vi "Main VI.vi"(11 "Error In":errorcluster) -> (15 "Error Out":errorcluster)   [LabVIEW 2020, in "DNL INL Test.lvlib"]
uses:
  DNL INL Test.lvlib
  Typedef/Queue Operation.ctl
  Typedef/Data Line.ctl
  Class/INL DNL Test/Test/Parent/Test.lvclass
  Typedef/User event controls.ctl
  Class/INL DNL Test/Test/Children/INL DNL Test/INL DNL Test.lvclass
  D:/SDLC/Class/INL DNL Test/Test/Parent/Test.lvclass
  Class/INL DNL Test/Device/Parent/Device.lvclass
panel:
  in  "Calculate":bool
  in  "Available Test":string(tree)
  out "Graph Pic":picture
  out "Config Pic":picture
  out "Mode Pic":picture
  out "Home Pic":picture
  in  "Status and graph":bool
  in  "Configuration":bool
  in  "Mode selection":bool
  in  "Home":bool
  out "Status":string
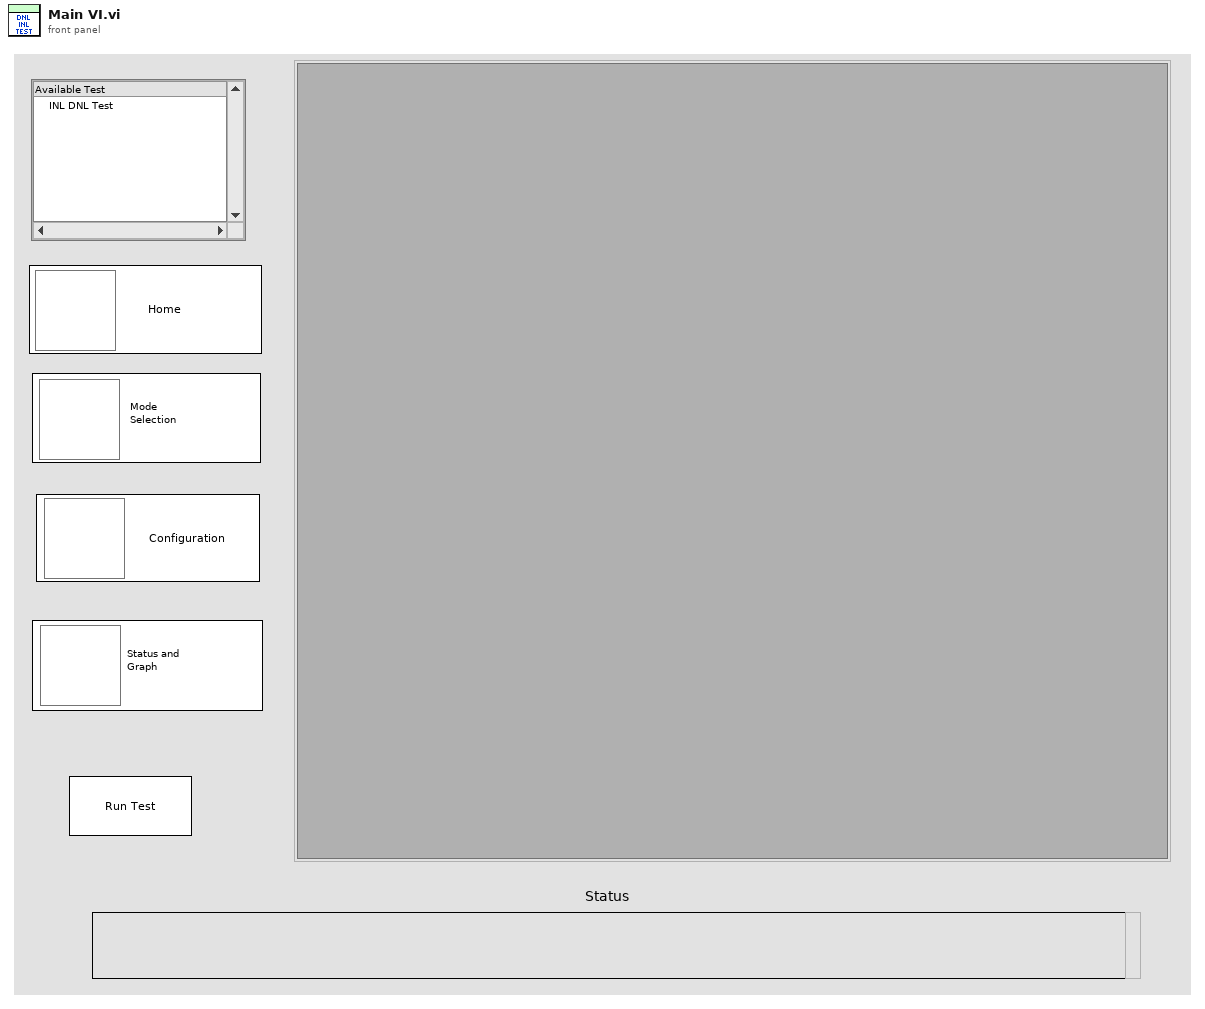
[diagram p1: front panel]
types:
  T1 = typedef "DNL INL Test.lvlib/Data Line.ctl" = cluster{"DVR":refnum<data-value>, "Subpanel Ref":refnum<vi>, "Class Selected?":bool, "Status Msg":string, "Test Name":string, "Status":string, "Mode Ref":refnum<vi>, "Config Ref":refnum<vi>}
  T2 = typedef "DNL INL Test.lvlib/Queue Operation.ctl" = enum16{"Create Queue", "Enqueue", "Dequeue", "Enstack", "Flush Queue", "Release Queue"}
  T3 = typedef "DNL INL Test.lvlib/User event controls.ctl" = enum16{"Create", "Generate", "Get Ref", "Destroy"}
  T4 = typedef "imagedata.ctl" = cluster{"image type":i32, "image depth":i32, "image":u8[], "mask":u8[], "colors":u32[], "Rectangle":cluster{"left":i16, "top":i16, "right":i16, "bottom":i16}}
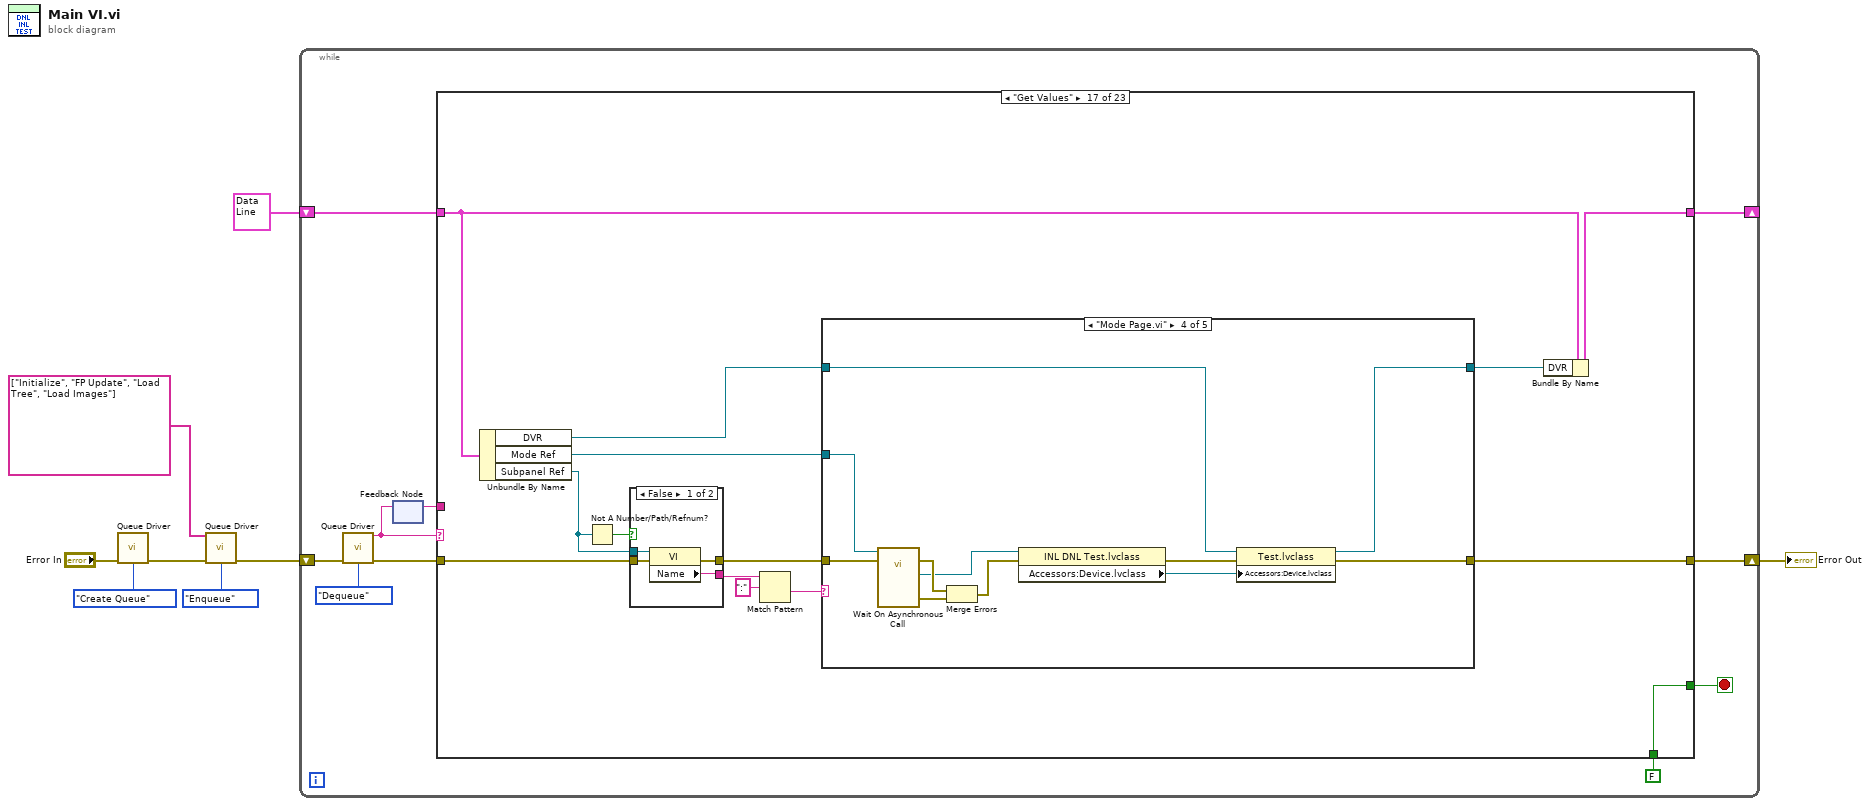
[diagram p0: block diagram]
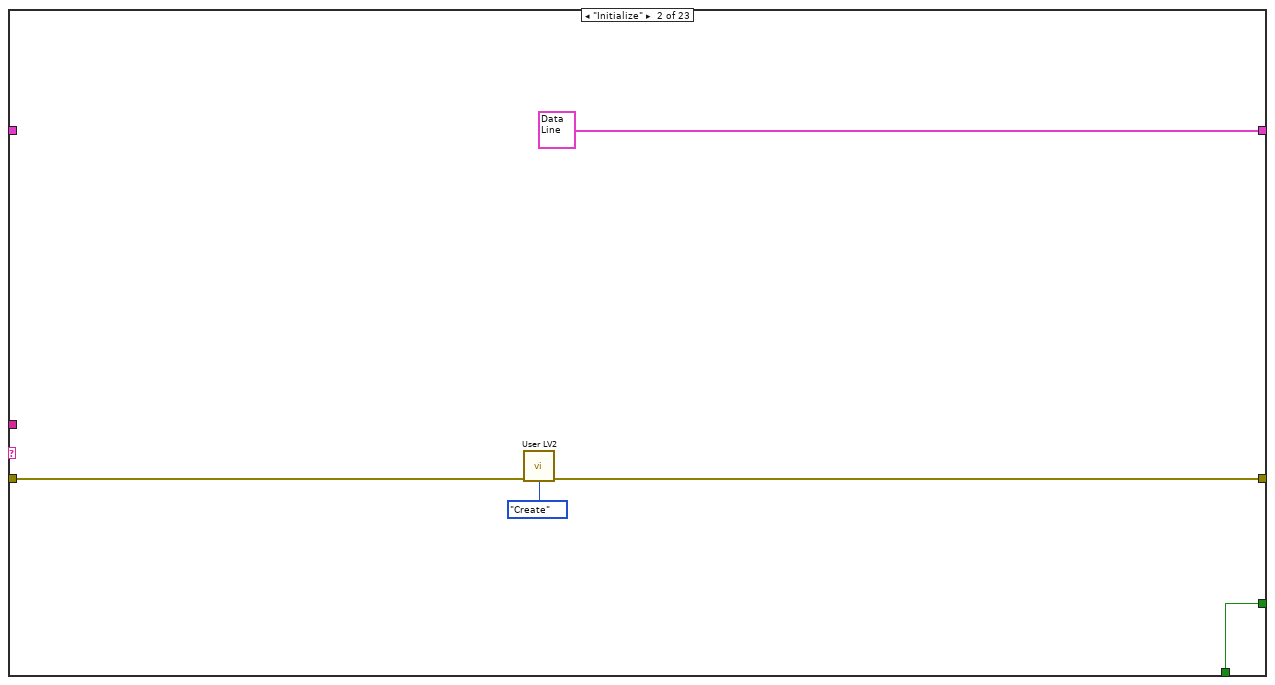
[diagram p3: hidden frame]
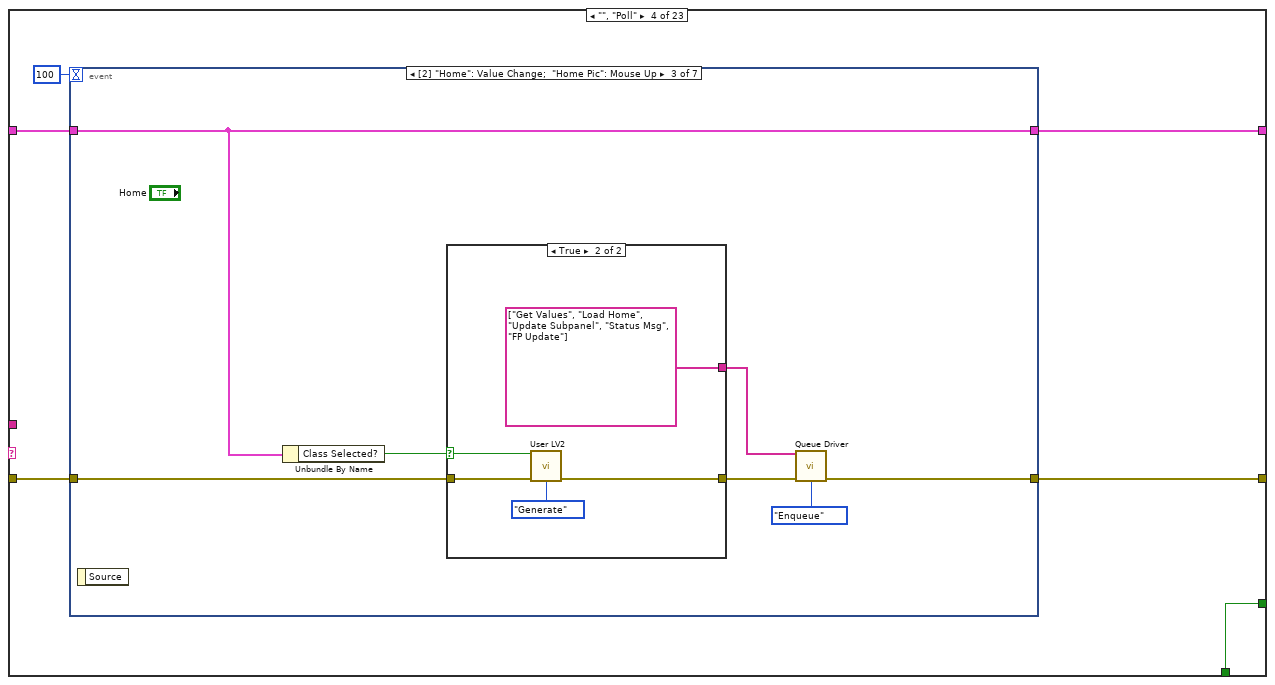
[diagram p5: hidden frame]
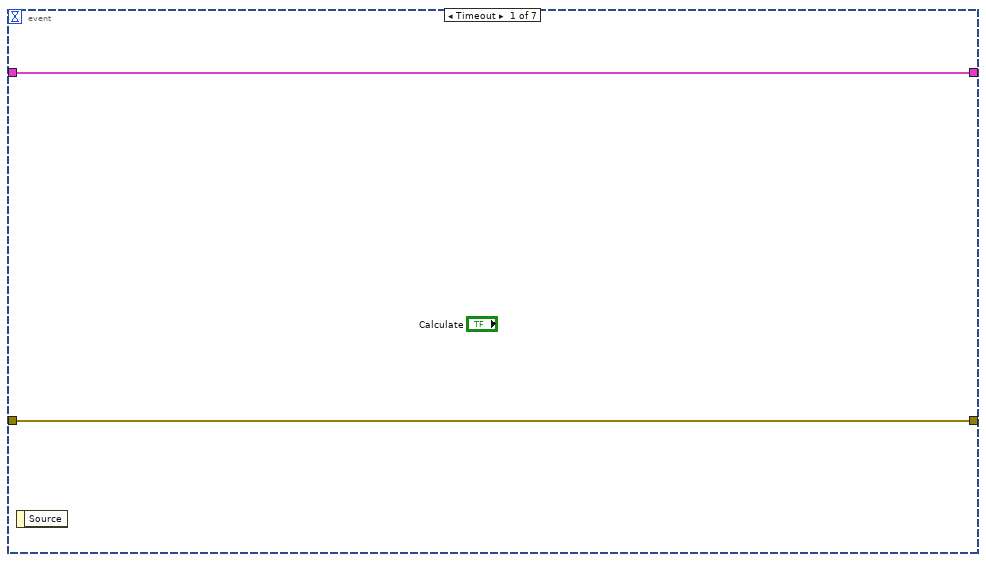
[diagram p6: hidden frame]
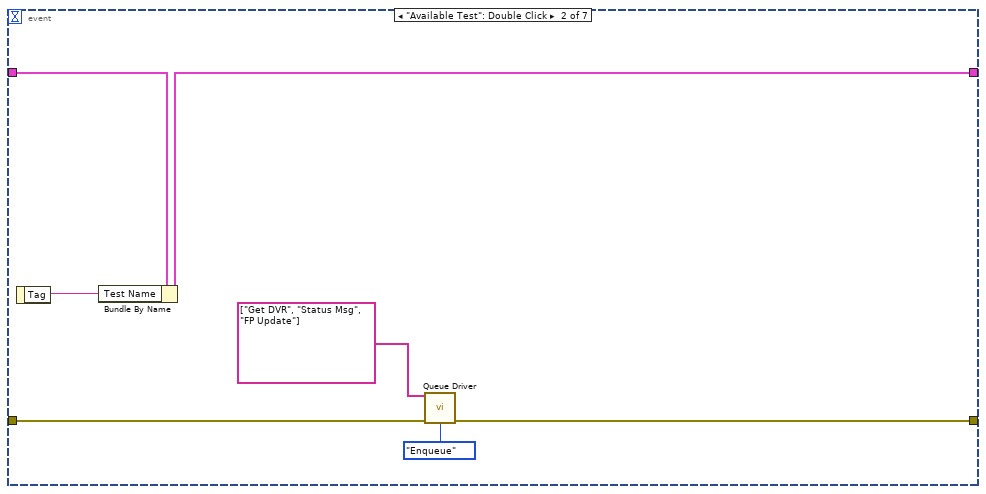
[diagram p7: hidden frame]
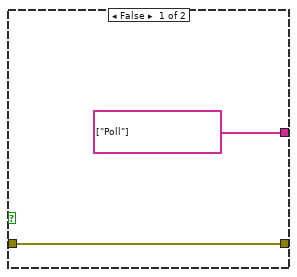
[diagram p8: hidden frame]
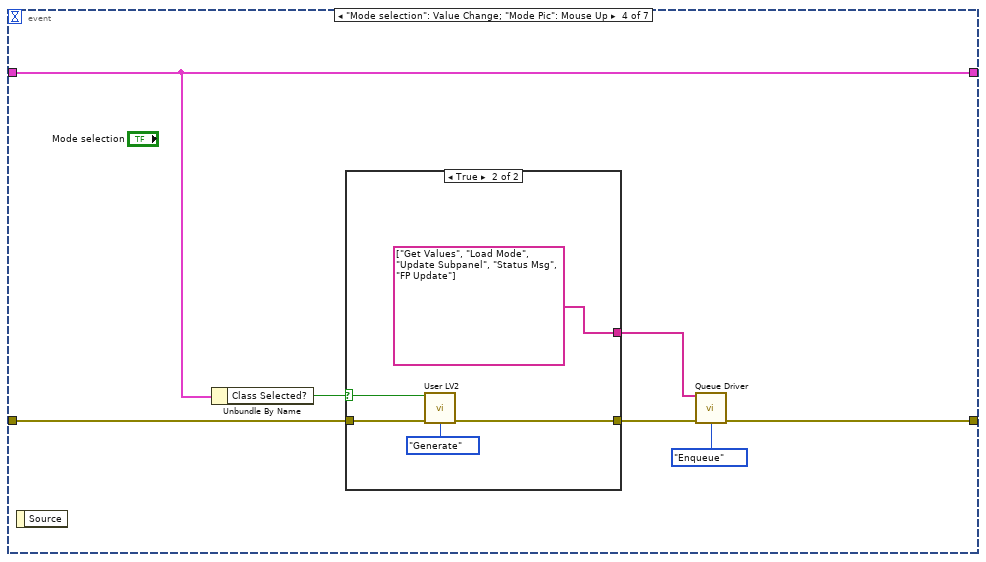
[diagram p9: hidden frame]
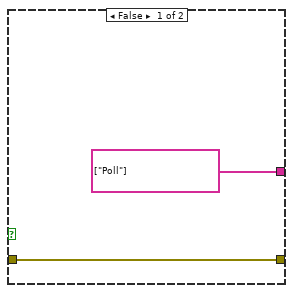
[diagram p10: hidden frame]
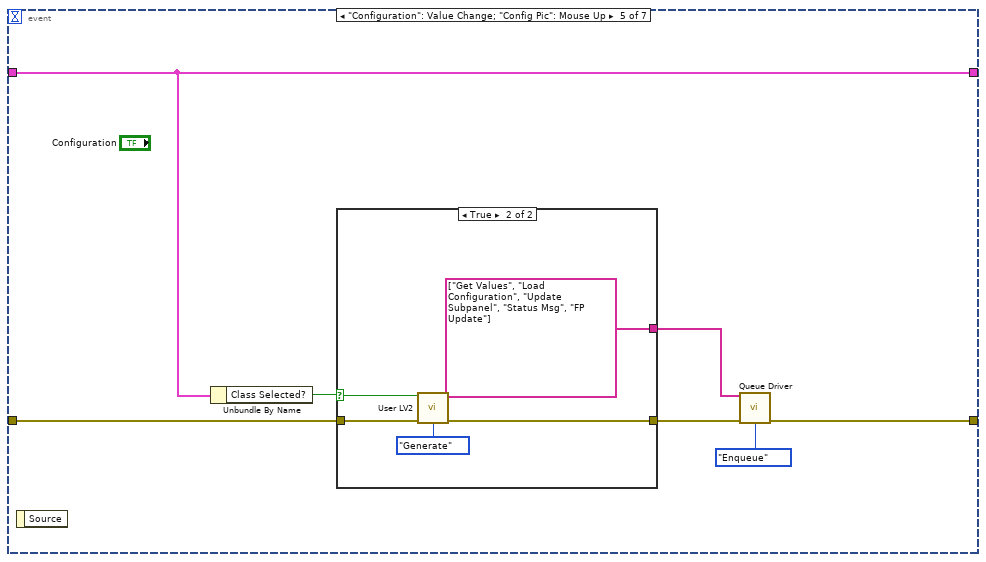
[diagram p11: hidden frame]
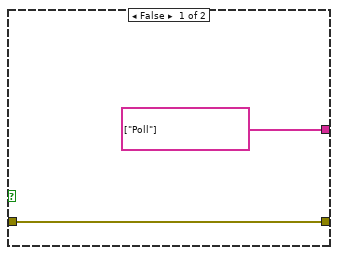
[diagram p12: hidden frame]
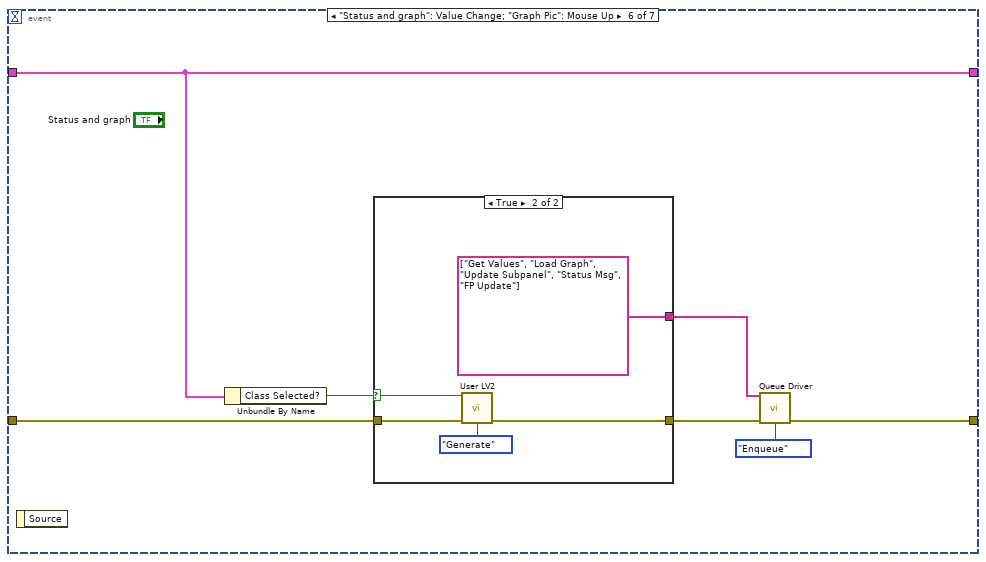
[diagram p13: hidden frame]
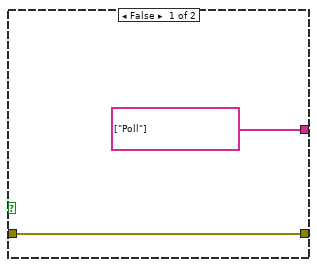
[diagram p14: hidden frame]
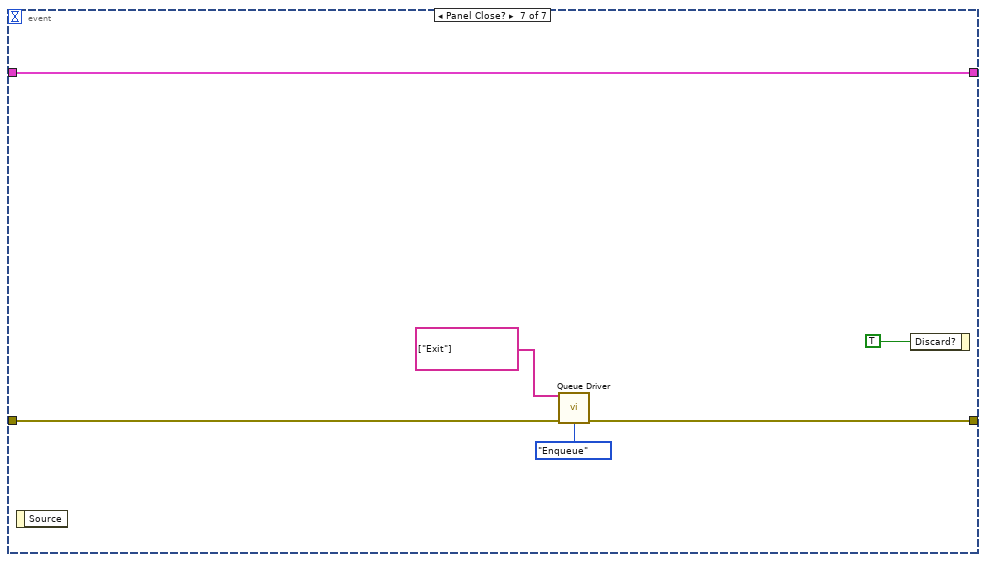
[diagram p15: hidden frame]
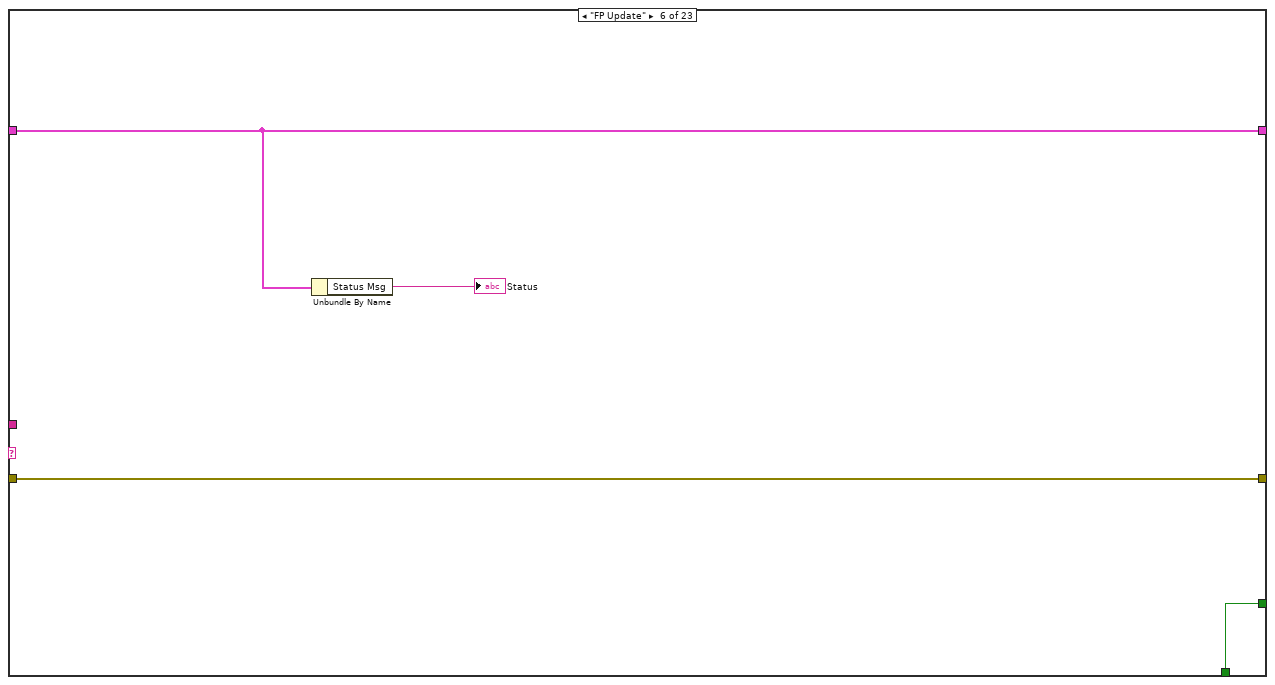
[diagram p17: hidden frame]
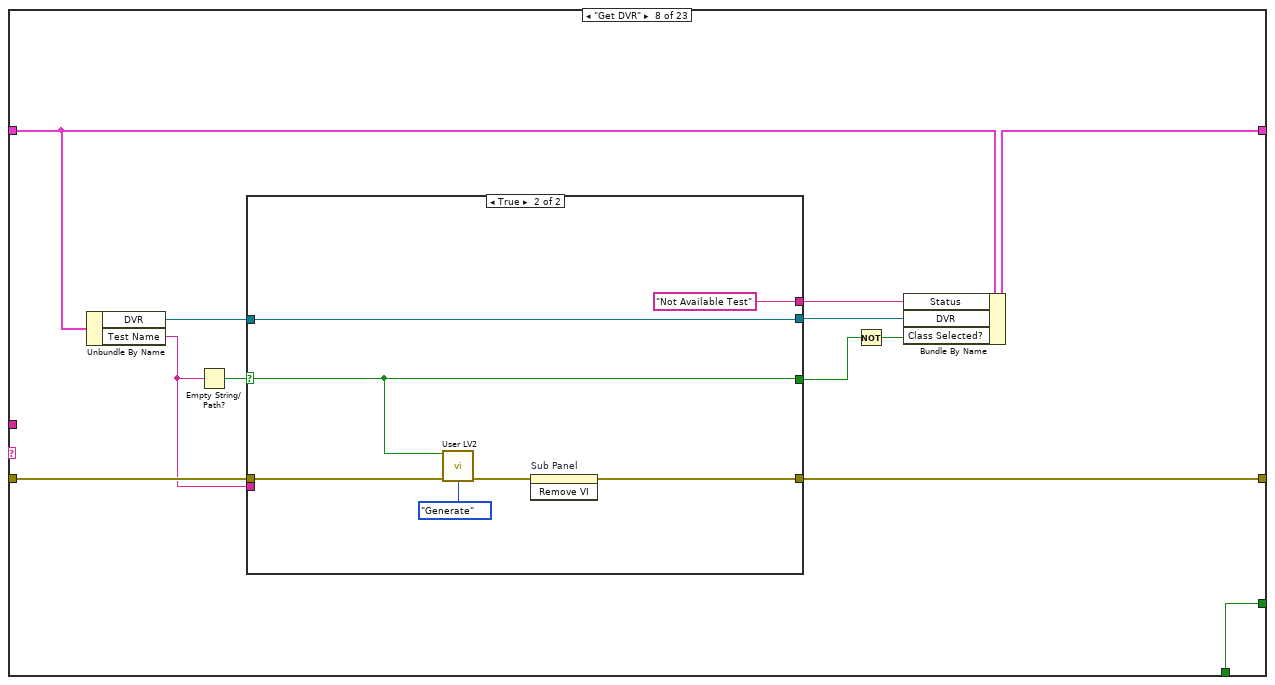
[diagram p19: hidden frame]
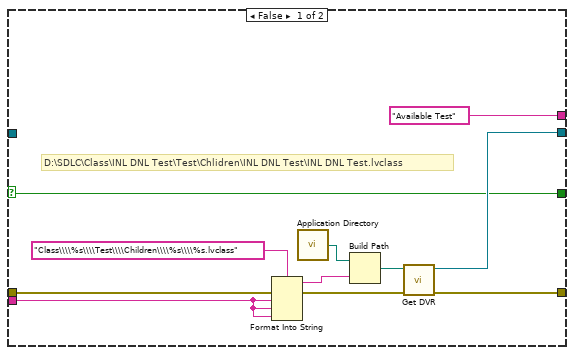
[diagram p20: hidden frame]
diagram:
  n1 = call "Queue Driver.vi"("Error In"="Error In", "Queue Operation"=Queue_Operation."Create Queue") -> ("Error Out"=w6:errorcluster)  [unwired: 12 in, 1 out]
  n2 = call "Queue Driver.vi"("States"=string[] ["Initialize", "FP Update", "Load Tree", "Load Images"], "Error In"=w6, "Queue Operation"=Queue_Operation."Enqueue") -> ("Error Out"=w3:errorcluster)  [unwired: 11 in, 1 out]
  n3 = while {
    shift-right: [w13] -> w2
    shift-left: w3 -> [w18]
    shift-right: [w9] -> _
    shift-left: T1 {"DVR"=refnum, "Subpanel Ref"=refnum, "Class Selected?"=FALSE, "Status Msg"="", "Test Name"="", "Status"="", "Mode Ref"=refnum, "Config Ref"=refnum} ("Data Line") -> [w10]
    stop <- w11 stop-if-true
    n4 = call "Queue Driver.vi"("Error In"=w18, "Queue Operation"=Queue_Operation."Dequeue") -> ("Dequeue Element"=w16:string, "Error Out"=w14:errorcluster)  [unwired: 12 in]
    n5 = feedback-in #1(w16) -> ()
    n6 = feedback #1() -> (w15:string)  [unwired: 1 in]
    n7 = case shown="\"Get Values\"" w16 {
      selector: w16 -> [_ _ _ _ _ _ _ _ _ _ _ _ _ _ _ _ _ _ _ _ _ _ w378]
      tunnel: w15 -> [_ _ _ _ _ _ _ _ _ _ _ _ _ _ _ _ _ _ w342 _ _ _ _]
      tunnel: w14 -> [w21 w26 w29 w35 w109 w113 w116 w127 w153 w182 w184 w200 w209 w219 w224 w233 w296 w325 w345 w348 w364 w367 w381]
      tunnel: [w21 w24 w29 w34 w109 w113 w116 w126 w151 w182 w190 w193 w208 w214 w221 w232 w295 w325 w332 w348 w360 w367 w369] -> w13
      tunnel: FALSE -> [w20 w25 w28 w32 w108 w112 w115 w128 w158 w181 w191 w201 w211 w220 w225 w234 w297 w324 w326 w347 _ w366 w382]
      tunnel: [w20 w25 w28 w32 w108 w112 w115 w128 w158 w181 w191 w201 w211 w220 w225 w234 w297 w324 w326 w347 TRUE ("T button?") w366 w382] -> w11
      tunnel: w10 -> [w19 _ w27 w31 w107 w111 w114 w121 w157 w180 w188 w198 w207 w217 w223 w228 w286 w323 w329 w346 w353 w365 w368]
      tunnel: [w19 T1 {"DVR"=refnum, "Subpanel Ref"=refnum, "Class Selected?"=FALSE, "Status Msg"="", "Test Name"="", "Status"="", "Mode Ref"=refnum, "Config Ref"=refnum} ("Data Line") w27 w30 w107 w111 w114 w120 w157 w180 w185 w196 w204 w213 w223 w226 w284 w323 w327 w346 w353 w365 w368] -> w9
      frame "/****Initialize****/" {
      }
      frame "Initialize" {
        n8 = call "User LV2.vi"("Error In"=w26, "User event controls"=User_event_controls."Create") -> ("Error Out"=w24:errorcluster)  [unwired: 12 in, 1 out]
      }
      frame "/****User inputs****/" {
      }
      frame "", "Poll" {
        n9 = event shown="[2] \"Home\": Value Change;  \"Home Pic\": Mouse Up" {
          selector: _ -> [_ _ _ _ _ _ _]
          dyn-events: _ -> [_ _ _ _ _ _ _]
          timeout: 100 -> [_ _ _ _ _ _ _]
          tunnel: w35 -> [w37 w41 w48 w62 w76 w90 w104]
          tunnel: [w37 w40 w51 w63 w77 w91 w103] -> w34
          tunnel: w31 -> [w36 w44 w46 w60 w74 w88 w106]
          tunnel: [w36 w43 w46 w60 w74 w88 w106] -> w30
          event Timeout {
            n10 = event-data() -> ()  [unwired: 1 in, 1 out]
          }
          event "Available Test": Double Click {
            n11 = event-data() -> ("Tag"=w42:string)  [unwired: 1 in]
            n12 = Bundle By Name(cluster=w44, "Test Name"=w42) -> (w43:T1)
            n13 = call "Queue Driver.vi"("States"=string[] ["Get DVR", "Status Msg", "FP Update"], "Error In"=w41, "Queue Operation"=Queue_Operation."Enqueue") -> ("Error Out"=w40:errorcluster)  [unwired: 11 in, 1 out]
          }
          event "Home": Value Change; "Home Pic": Mouse Up {
            n14 = event-data() -> ()  [unwired: 1 in, 1 out]
            n15 = Unbundle By Name(w46) -> ("Class Selected?"=w45:bool)
            n16 = case shown="True" w45 {
              selector: w45 -> [_ w54]
              tunnel: [string[] ["Poll"] ("States") string[] ["Get Values", "Load Home", "Update Subpanel", "Status Msg", "FP Update"] ("States")] -> w49
              tunnel: w48 -> [w52 w57]
              tunnel: [w52 w56] -> w47
              frame False {
              }
              frame True {
                n17 = call "User LV2.vi"("Stop"=w54, "Error In"=w57, "User event controls"=User_event_controls."Generate") -> ("Error Out"=w56:errorcluster)  [unwired: 11 in, 1 out]
              }
            }
            n18 = call "Queue Driver.vi"("States"=w49, "Error In"=w47, "Queue Operation"=Queue_Operation."Enqueue") -> ("Error Out"=w51:errorcluster)  [unwired: 11 in, 1 out]
          }
          event "Mode selection": Value Change; "Mode Pic": Mouse Up {
            n19 = event-data() -> ()  [unwired: 1 in, 1 out]
            n20 = Unbundle By Name(w60) -> ("Class Selected?"=w59:bool)
            n21 = case shown="True" w59 {
              selector: w59 -> [_ w68]
              tunnel: [string[] ["Poll"] ("States") string[] ["Get Values", "Load Mode", "Update Subpanel", "Status Msg", "FP Update"] ("States")] -> w64
              tunnel: [w66 w70] -> w61
              tunnel: w62 -> [w66 w72]
              frame False {
              }
              frame True {
                n22 = call "User LV2.vi"("Stop"=w68, "Error In"=w72, "User event controls"=User_event_controls."Generate") -> ("Error Out"=w70:errorcluster)  [unwired: 11 in, 1 out]
              }
            }
            n23 = call "Queue Driver.vi"("States"=w64, "Error In"=w61, "Queue Operation"=Queue_Operation."Enqueue") -> ("Error Out"=w63:errorcluster)  [unwired: 11 in, 1 out]
          }
          event "Configuration": Value Change; "Config Pic": Mouse Up {
            n24 = event-data() -> ()  [unwired: 1 in, 1 out]
            n25 = Unbundle By Name(w74) -> ("Class Selected?"=w73:bool)
            n26 = case shown="True" w73 {
              selector: w73 -> [_ w82]
              tunnel: [string[] ["Poll"] ("States") string[] ["Get Values", "Load Configuration", "Update Subpanel", "Status Msg", "FP Update"] ("States")] -> w78
              tunnel: w76 -> [w80 w86]
              tunnel: [w80 w84] -> w75
              frame False {
              }
              frame True {
                n27 = call "User LV2.vi"("Stop"=w82, "Error In"=w86, "User event controls"=User_event_controls."Generate") -> ("Error Out"=w84:errorcluster)  [unwired: 11 in, 1 out]
              }
            }
            n28 = call "Queue Driver.vi"("States"=w78, "Error In"=w75, "Queue Operation"=Queue_Operation."Enqueue") -> ("Error Out"=w77:errorcluster)  [unwired: 11 in, 1 out]
          }
          event "Status and graph": Value Change; "Graph Pic": Mouse Up {
            n29 = event-data() -> ()  [unwired: 1 in, 1 out]
            n30 = Unbundle By Name(w88) -> ("Class Selected?"=w87:bool)
            n31 = case shown="True" w87 {
              selector: w87 -> [_ w96]
              tunnel: [string[] ["Poll"] ("States") string[] ["Get Values", "Load Graph", "Update Subpanel", "Status Msg", "FP Update"] ("States")] -> w92
              tunnel: [w94 w98] -> w89
              tunnel: w90 -> [w94 w100]
              frame False {
              }
              frame True {
                n32 = call "User LV2.vi"("Stop"=w96, "Error In"=w100, "User event controls"=User_event_controls."Generate") -> ("Error Out"=w98:errorcluster)  [unwired: 11 in, 1 out]
              }
            }
            n33 = call "Queue Driver.vi"("States"=w92, "Error In"=w89, "Queue Operation"=Queue_Operation."Enqueue") -> ("Error Out"=w91:errorcluster)  [unwired: 11 in, 1 out]
          }
          event Panel Close? {
            n34 = event-data() -> ()  [unwired: 1 in, 1 out]
            n35 = call "Queue Driver.vi"("States"=string[] ["Exit"], "Error In"=w104, "Queue Operation"=Queue_Operation."Enqueue") -> ("Error Out"=w103:errorcluster)  [unwired: 11 in, 1 out]
            n36 = event-data("Discard?"=TRUE) -> ()  [unwired: 1 in, 1 out]
          }
        }
      }
      frame "/****Front panel updates****/" {
      }
      frame "FP Update" {
        n37 = Unbundle By Name(w111) -> ("Status Msg"=→"Status":string)
      }
      frame "/****Functionality****/" {
      }
      frame "Get DVR" {
        n38 = Unbundle By Name(w121) -> ("DVR"=w125:refnum<data-value>, "Test Name"=w124:string)
        n39 = Empty String/Path?(string/path=w124) -> (empty?=w123:bool)
        n40 = case shown="True" w123 {
          selector: w123 -> [w130 w140]
          tunnel: w127 -> [w139 w146]
          tunnel: [w134 w144] -> w126
          tunnel: w124 -> [w132 _]
          tunnel: [w133 w143] -> w119
          tunnel: w125 -> [_ w143]
          tunnel: [w130 w140] -> w118
          tunnel: ["Available Test" ("Status") "Not Available Test" ("Status")] -> w117
          frame False {
            # "D:\\SDLC\\Class\\INL DNL Test\\Test\\Chlidren\\INL DNL Test\\INL DNL Test.lvclass"
            n41 = Format Into String(format string="Class\\\\%s\\\\Test\\\\Children\\\\%s\\\\%s.lvclass", error in=w139, w132, w132, w132) -> (resulting string=w136:string, error out=w135:errorcluster)  [unwired: 1 in]
            n42 = call <vilib>:"Application Directory.vi"() -> ("Application Directory"=w137:path)
            n43 = Build Path(base path=w137, name or relative path=w136) -> (appended path=w131:path)
            n44 = call "Get DVR.vi"("Error in"=w135, "Class path"=w131) -> ("Error out"=w134:errorcluster, "DVR Out"=w133:refnum<data-value>)  [unwired: 8 in]
          }
          frame True {
            n45 = call "User LV2.vi"("Stop"=w140, "Error In"=w146, "User event controls"=User_event_controls."Generate") -> ("Error Out"=w142:errorcluster)  [unwired: 11 in, 1 out]
            n46 = invoke on="Sub Panel" class="SubPnl" method="Remove VI"(error in=w142) -> (error out=w144:errorcluster)  [unwired: 2 in, 2 out]
          }
        }
        n47 = Not(x=w118) -> (.not. x?=w122:bool)
        n48 = Bundle By Name(cluster=w121, "Status"=w117, "DVR"=w119, "Class Selected?"=w122) -> (w120:T1)
      }
      frame "Load Tree" {
        n49 = invoke on="Available Test" class="Tree (strict)" method="Edit Tree Items.Delete"(error in=w153, "tag"="", "Delete Children"=TRUE ("Delete Children?")) -> (error out=w149:errorcluster)  [unwired: 2 in, 4 out]
        n50 = call <vilib>:"Application Directory.vi"() -> ("Application Directory"=w156:path)
        n51 = Build Path(base path=w156, name or relative path=path "Class") -> (appended path=w154:path)
        n52 = List Folder(path=w154, error in=w149) -> (folder names=w150:string[], error out=w152:errorcluster)  [unwired: 2 in, 2 out]
        n53 = for {
          shift-right: [w161] -> w151
          shift-left: w152 -> [w162]
          tunnel: w150 -> [w159] mode=indexing
          n54 = invoke on="Available Test" class="Tree (strict)" method="Edit Tree Items.Add Item"(error in=w162, "Parent Tag"="", "Left Cell"=w159, "Child Tag"=w159) -> (error out=w161:errorcluster)  [unwired: 5 in, 8 out]
        }
      }
      frame "Load Images" {
        n55 = call <vilib>:"Application Directory.vi"() -> ("Application Directory"=w163:path)
        n56 = Build Path(base path=w163, name or relative path=path "Images/Home.png") -> (appended path=w177:path)
        n57 = Build Path(base path=w163, name or relative path=path "Images/Mode Selection.png") -> (appended path=w176:path)
        n58 = Build Path(base path=w163, name or relative path=path "Images/Configuration.png") -> (appended path=w170:path)
        n59 = Build Path(base path=w163, name or relative path=path "Images/Status and Graph.png") -> (appended path=w167:path)
        n60 = call <vilib>:"Read PNG File.vi"("path to PNG file"=w177) -> ("image data"=w179:T4)  [unwired: 8 in, 2 out]
        n61 = call <vilib>:"Read PNG File.vi"("path to PNG file"=w176) -> ("image data"=w175:T4)  [unwired: 8 in, 2 out]
        n62 = call <vilib>:"Read PNG File.vi"("path to PNG file"=w170) -> ("image data"=w171:T4)  [unwired: 8 in, 2 out]
        n63 = call <vilib>:"Read PNG File.vi"("path to PNG file"=w167) -> ("image data"=w168:T4)  [unwired: 8 in, 2 out]
        n64 = call <vilib>:"Draw Flattened Pixmap.vi"("image data"=w179) -> ("new picture"=→"Home Pic":picture)  [unwired: 8 in]
        n65 = call <vilib>:"Draw Flattened Pixmap.vi"("image data"=w175) -> ("new picture"=→"Mode Pic":picture)  [unwired: 8 in]
        n66 = call <vilib>:"Draw Flattened Pixmap.vi"("image data"=w171) -> ("new picture"=→"Config Pic":picture)  [unwired: 8 in]
        n67 = call <vilib>:"Draw Flattened Pixmap.vi"("image data"=w168) -> ("new picture"=→"Graph Pic":picture)  [unwired: 8 in]
      }
      frame "Load Home" {
        n68 = Unbundle By Name(w188) -> ("DVR"=w189:refnum<data-value>)
        n69 = call "Home_Ref_API.vi"("DVR In"=w189, "Error In"=w184) -> ("DVR Out"=w187:refnum<data-value>, "VI Ref"=w186:refnum<vi>, "Error Out"=w190:errorcluster)  [unwired: 10 in, 1 out]
        n70 = Bundle By Name(cluster=w188, "Status"="Home", "DVR"=w187, "Subpanel Ref"=w186) -> (w185:T1)
      }
      frame "Load Mode" {
        n71 = Unbundle By Name(w198) -> ("DVR"=w199:refnum<data-value>)
        n72 = call "Mode_Ref_API.vi"("DVR In"=w199, "Error In"=w200) -> ("DVR Out"=w197:refnum<data-value>, "VI Ref"=w194:refnum<vi>, "Mode Ref"=w192:refnum<vi>, "Error out"=w193:errorcluster)  [unwired: 10 in]
        n73 = Bundle By Name(cluster=w198, "Status"="Mode", "DVR"=w197, "Subpanel Ref"=w194, "Mode Ref"=w192) -> (w196:T1)
      }
      frame "Load Configuration" {
        n74 = Unbundle By Name(w207) -> ("DVR"=w210:refnum<data-value>)
        n75 = call "Configuration_Ref_API.vi"("DVR In"=w210, "Error In"=w209) -> ("DVR Out"=w206:refnum<data-value>, "VI Ref"=w205:refnum<vi>, "Configuration Ref"=w202:refnum<vi>, "Error Out"=w208:errorcluster)  [unwired: 10 in]
        n76 = Bundle By Name(cluster=w207, "Status"="Configuration", "DVR"=w206, "Subpanel Ref"=w205, "Config Ref"=w202) -> (w204:T1)
      }
      frame "Load Graph" {
        n77 = Unbundle By Name(w217) -> ("DVR"=w218:refnum<data-value>)
        n78 = call "Status_Ref_API.vi"("DVR In"=w218, "Error In"=w219) -> ("DVR Out"=w216:refnum<data-value>, "Status Ref"=w215:refnum<vi>, "Error Out"=w214:errorcluster)  [unwired: 11 in]
        n79 = Bundle By Name(cluster=w217, "Status"="Graph", "DVR"=w216, "Subpanel Ref"=w215) -> (w213:T1)
      }
      frame "Update Subpanel" {
        n80 = Unbundle By Name(w223) -> ("Subpanel Ref"=w222:refnum<vi>)
        n81 = invoke on="Sub Panel" class="SubPnl" method="Insert VI"(error in=w224, "VI Ref"=w222) -> (error out=w221:errorcluster)  [unwired: 2 in, 3 out]
      }
      frame "Status Msg" {
        n82 = Unbundle By Name(w228) -> ("Status"=w231:string, "Test Name"=w230:string, "Status Msg"=w229:string)
        n83 = case shown="\"Error\"" w231 {
          tunnel: w233 -> [w240 w246 w252 w258 w264 w270 w276 w283]
          tunnel: [w239 w245 w251 w257 w263 w269 w275 w282] -> w232
          tunnel: w230 -> [_ _ _ _ _ _ _ w280]
          tunnel: w229 -> [w236 w242 w248 w254 w260 w266 w272 w278]
          tunnel: [w235 w241 w247 w253 w259 w265 w271 w277] -> w227
          frame "Not Available Test" {
            n84 = Format Into String(format string=" Select the available tests. %s%s", error in=w240, "\r", w236) -> (resulting string=w235:string, error out=w239:errorcluster)  [unwired: 1 in]
          }
          frame "Home" {
            n85 = Format Into String(format string=" Home Page is laoded for the test. %s%s", error in=w246, "\r", w242) -> (resulting string=w241:string, error out=w245:errorcluster)  [unwired: 1 in]
          }
          frame "Mode" {
            n86 = Format Into String(format string="Available Modes for the test is displayed. %s%s", error in=w252, "\r", w248) -> (resulting string=w247:string, error out=w251:errorcluster)  [unwired: 1 in]
          }
          frame "Configuration" {
            n87 = Format Into String(format string="Available Configuration/Settings for the test is displayed. %s%s", error in=w258, "\r", w254) -> (resulting string=w253:string, error out=w257:errorcluster)  [unwired: 1 in]
          }
          frame "Graph" {
            n88 = Format Into String(format string=" Result page to plot/show data is displayed. %s%s", error in=w264, "\r", w260) -> (resulting string=w259:string, error out=w263:errorcluster)  [unwired: 1 in]
          }
          frame "Error" {
            n89 = Format Into String(format string=" Error Occured!!!  %s%s", error in=w270, "\r", w266) -> (resulting string=w265:string, error out=w269:errorcluster)  [unwired: 1 in]
          }
          frame Default {
            n90 = Format Into String(format string=" Unknown status %s%s", error in=w276, "\r", w272) -> (resulting string=w271:string, error out=w275:errorcluster)  [unwired: 1 in]
          }
          frame "Available Test" {
            n91 = Format Into String(format string=" \"%s\" is selected %s%s", error in=w283, w280, "\r", w278) -> (resulting string=w277:string, error out=w282:errorcluster)  [unwired: 1 in]
          }
        }
        n92 = Bundle By Name(cluster=w228, "Status Msg"=w227) -> (w226:T1)
      }
      frame "Get Values" {
        n93 = Unbundle By Name(w286) -> ("DVR"=w288:refnum<data-value>, "Mode Ref"=w287:refnum<vi>, "Subpanel Ref"=w289:refnum<vi>)
        n94 = Not A Number/Path/Refnum?(number/path/refnum=w289) -> (NaN/Path/Refnum?=w293:bool)
        n95 = case shown="False" w293 {
          tunnel: w296 -> [w301 w303]
          tunnel: [w300 w303] -> w294
          tunnel: [w299 "Default" ("Name")] -> w292
          tunnel: w289 -> [w298 _]
          frame False {
            n96 = property class="VI"(reference=w298, error in=w301) -> (error out=w300:errorcluster, "Name"=w299:string)  [unwired: 1 out]
          }
          frame True {
          }
        }
        n97 = Match Pattern(string=w292, regular expression=":") -> (after substring=w290:string)  [unwired: 1 in, 3 out]
        n98 = case shown="\"Mode Page.vi\"" w290 {
          tunnel: w294 -> [w305 w307 w309 w320 w321]
          tunnel: [w305 w307 w309 w315 w321] -> w295
          tunnel: w288 -> [w304 w306 w308 w314 w322]
          tunnel: [w304 w306 w308 w311 w322] -> w285
          tunnel: w287 -> [_ _ _ w319 _]
          frame "Home Page.vi" {
          }
          frame "Configuration Page.vi" {
          }
          frame "Status Page.vi" {
          }
          frame "Mode Page.vi" {
            n99 = call-by-ref "Wait On Asynchronous Call"(reference=w319, error in=w320) -> (error out=w318:errorcluster, "Error out"=w317:errorcluster, "INL DNL Test out"=w312:refnum<class "INL DNL Test.lvclass">)  [unwired: 10 in, 1 out]
            n100 = Merge Errors(w318, w317) -> (w316:errorcluster)
            n101 = property class="INL DNL Test.lvclass"(reference=w312, error in=w316) -> (error out=w313:errorcluster, "Accessors:Device.lvclass"=w310:refnum<class "Device.lvclass">)  [unwired: 1 out]
            n102 = property class="Test.lvclass"(reference=w314, error in=w313, "Accessors:Device.lvclass"=w310) -> (reference out=w311:refnum<data-value>, error out=w315:errorcluster)
          }
          frame Default {
          }
        }
        n103 = Bundle By Name(cluster=w286, "DVR"=w285) -> (w284:T1)
      }
      frame "/****Error****/" {
      }
      frame "Error" {
        n104 = Unbundle By Name(w345) -> ("code"=w341:i32, "source"=w340:string)
        n105 = call <vilib>:"Clear Errors.vi"("error in (no error)"=w345, "specific error code to clear (0: all)"=w341) -> ("error out"=w344:errorcluster)  [unwired: 4 in, 1 out]
        n106 = Format Into String(format string="Error Occurred in \"%s\" State \n\nError Code: %d\nDescription: %s\n\nDo you want to stop or continue? \n", error in=w344, w342, w341, w340) -> (resulting string=w339:string, error out=w333:errorcluster)  [unwired: 1 in]
        n107 = Two Button Dialog(message=w339, 1:"Continue" ("F button name (\"Cancel\")"), 2:"Stop" ("T button name (\"OK\")")) -> (T button?=w336:bool)
        n108 = Select(t=string[] ["Exit", "FP Update", "Status Msg"] ("States"), s=w336, f=string[] ["FP Update", "Status Msg"] ("States")) -> (s? t:f=w330:string[])
        n109 = Bundle By Name(cluster=w329, "Status"="Error") -> (w327:T1)
        n110 = call "Queue Driver.vi"("States"=w330, "Error In"=w333, "Queue Operation"=Queue_Operation."Enstack") -> ("Error Out"=w332:errorcluster)  [unwired: 11 in, 1 out]
      }
      frame "/****Exit****/" {
      }
      frame "Exit" {
        n111 = Unbundle By Name(w353) -> ("DVR"=w352:refnum<data-value>, "Subpanel Ref"=w349:refnum<vi>)
        n112 = call "User LV2.vi"("Stop"=TRUE, "Error In"=w364, "User event controls"=User_event_controls."Generate") -> ("Error Out"=w357:errorcluster)  [unwired: 11 in, 1 out]
        n113 = call "User LV2.vi"("Error In"=w357, "User event controls"=User_event_controls."Destroy") -> ("Error Out"=w351:errorcluster)  [unwired: 12 in, 1 out]
        n114 = Close Reference(reference=w349, error in (no error)=w351) -> (error out=w350:errorcluster)
        n115 = call "Delete DVR.vi"("Error in"=w350, "DVR In"=w352) -> ("error out"=w354:errorcluster)  [unwired: 9 in]
        n116 = call "Queue Driver.vi"("Error In"=w354, "Queue Operation"=Queue_Operation."Flush Queue") -> ("Error Out"=w362:errorcluster)  [unwired: 12 in, 1 out]
        n117 = call "Queue Driver.vi"("Error In"=w362, "Queue Operation"=Queue_Operation."Release Queue") -> ("Error Out"=w360:errorcluster)  [unwired: 12 in, 1 out]
      }
      frame "/****Developer error****/" {
      }
      frame Default {
        n118 = Format Into String(format string="State name: %s\n\nState name not found\n\nDo you want to stop or continue?\n", error in=w381, w378) -> (resulting string=w377:string, error out=w380:errorcluster)  [unwired: 1 in]
        n119 = Two Button Dialog(message=w377, 1:"Continue" ("F button name (\"Cancel\")"), 2:"Stop" ("T button name (\"OK\")")) -> (T button?=w374:bool)
        n120 = Select(t=string[] ["Exit"] ("States"), s=w374, f=string[] ["Poll"] ("States")) -> (s? t:f=w371:string[])
        n121 = call "Queue Driver.vi"("States"=w371, "Error In"=w380, "Queue Operation"=Queue_Operation."Enqueue") -> ("Error Out"=w369:errorcluster)  [unwired: 11 in, 1 out]
      }
    }
  }
  "Error Out" <- w2
